vi "LVClass_Camera get Parameter Values OnlyGet.vi"(0 "Camera in":refnum<class "Camera.lvclass">, 11 "error in (no error)":errorcluster) -> (4 "Camera out":refnum<class "Camera.lvclass">, 6 "ListOfGettableValue":T1[](array[typedef]), 15 "error out":errorcluster)   [LabVIEW 2020, in "Camera.lvclass"]
doc: "Get camera parameters which are only gettable parameter \n\n<B>CameraIn</B> : Camera object.\n<B>CameraOut</B> : Camera object.\n<B>ListOfGettableValue</B> : Array of the parameter with readen value from camera object."
uses:
  Camera.lvclass
  CameraParametersSetup.ctl
  CameraParameters_Type.ctl
  Camera.lvclass/Camera.ctl
  LVClass_Camera Read acquisition state.vi
  LVClass_Camera Read all camera parameters.vi
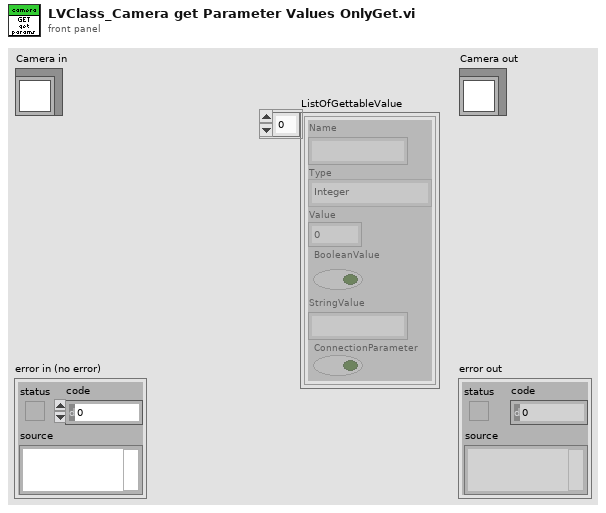
[diagram p1: front panel]
types:
  T1 = typedef "CameraParametersSetup.ctl" = cluster{"Name":string, "Type":T2, "Value":dbl, "BooleanValue":bool, "StringValue":string, "ConnectionParameter":bool}
  T2 = typedef "CameraParameters_Type.ctl" = enum16{"Integer", "Real", "String", "Boolean"}
  T3 = typedef "CameraAcquisitionState.ctl" = enum16{"Stop", "Live"}
  T4 = typedef "ParameterID.ctl" = cluster{"Name":string, "ConnectionParameter?":bool, "Type":T2, "Authorization":T5, "OnFlyAuthorization":T6, "StringValue":string, "Value":dbl, "Min":dbl, "Max":dbl, "BooleanValue":bool, "StringParameterList":string[]}
  T5 = typedef "CameraParameters_Authorization.ctl" = enum16{"Disable", "Gettable", "Settable - Gettable"}
  T6 = typedef "CameraParameters_OnFlyAuthorization.ctl" = enum16{"None", "Gettable", "Settable", "Settable - Gettable"}
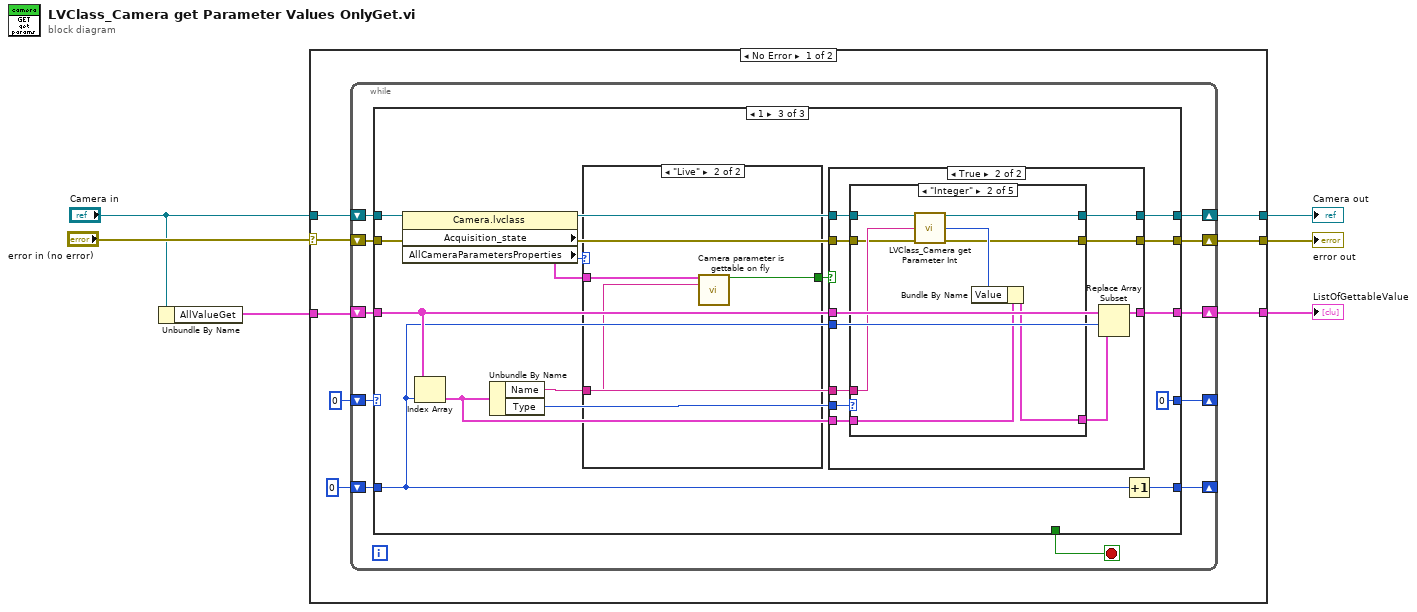
[diagram p0: block diagram]
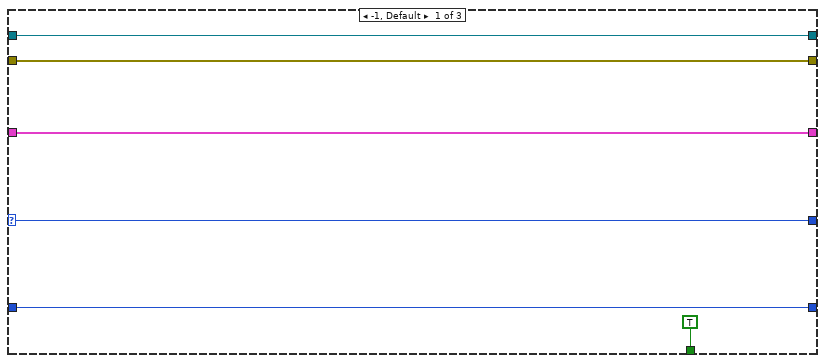
[diagram p2: hidden frame]
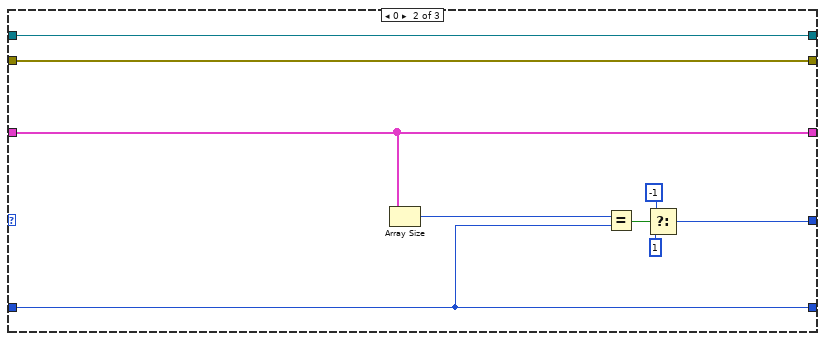
[diagram p3: hidden frame]
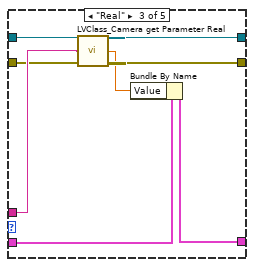
[diagram p6: hidden frame]
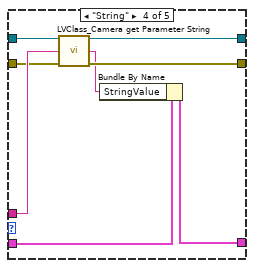
[diagram p7: hidden frame]
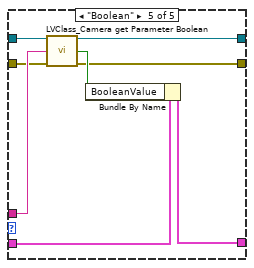
[diagram p8: hidden frame]
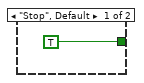
[diagram p9: hidden frame]
diagram:
  n1 = Unbundle By Name("Camera in") -> ("AllValueGet"=w1:T1[])
  n2 = case shown="No Error" "error in (no error)" {
    selector: "error in (no error)" -> [w10 w112]
    tunnel: [w11 w112] -> w5
    tunnel: [w12 w111] -> w4
    tunnel: "Camera in" -> [w14 w111]
    tunnel: [w9 _] -> w3
    tunnel: w1 -> [w7 _]
    frame No Error {
      n3 = while {
        shift-right: [w24] -> _
        shift-left: 0 -> [w23]
        shift-right: [w21] -> w11
        shift-left: w10 -> [w20]
        shift-right: [w22] -> w12
        shift-left: w14 -> [w25]
        shift-right: [w18] -> w9
        shift-left: w7 -> [w17]
        shift-right: [w15] -> _
        shift-left: 0 -> [w16]
        stop <- w19 stop-if-true
        n4 = case shown="1" w23 {
          selector: w23 -> [w26 _ _]
          tunnel: w25 -> [w30 w40 w48]
          tunnel: w20 -> [w29 w39 w46]
          tunnel: [w26 w33 0] -> w24
          tunnel: [w30 w40 w56] -> w22
          tunnel: [w29 w39 w55] -> w21
          tunnel: [TRUE _ _] -> w19
          tunnel: [w28 w38 w50] -> w18
          tunnel: w17 -> [w28 w38 w52]
          tunnel: w16 -> [w27 w36 w51]
          tunnel: [w27 w36 w54] -> w15
          frame -1, Default {
          }
          frame 0 {
            n5 = Array Size(array=w38) -> (size(s)=w37:i32)
            n6 = Equal?(x=w37, y=w36) -> (x = y?=w35:bool)
            n7 = Select(t=-1, s=w35, f=1) -> (s? t:f=w33:i32)
          }
          frame 1 {
            n8 = property class="Camera.lvclass"(reference=w48, error in=w46) -> (reference out=w47:refnum<class "Camera.lvclass">, error out=w45:errorcluster, "Acquisition_state"=w44:T3, "AllCameraParametersProperties"=w43:T4[])
            n9 = Index Array(array=w52, index=w51) -> (element=w53:T1)
            n10 = Unbundle By Name(w53) -> ("Name"=w41:string, "Type"=w49:T2)
            n11 = case shown="\"Live\"" w44 {
              tunnel: w43 -> [_ w109]
              tunnel: [TRUE w110] -> w42
              tunnel: w41 -> [_ w108]
              frame "Stop", Default {
              }
              frame "Live" {
                n12 = call "Camera parameter is gettable on fly.vi"("AllCameraParameters"=w109, "Name"=w108) -> ("Gettable?"=w110:bool)  [unwired: 13 in]
              }
            }
            n13 = case shown="True" w42 {
              tunnel: [w60 w71] -> w56
              tunnel: [w59 w70] -> w55
              tunnel: w53 -> [_ w69]
              tunnel: w52 -> [w58 w68]
              tunnel: w51 -> [_ w67]
              tunnel: [w58 w66] -> w50
              tunnel: w49 -> [_ w65]
              tunnel: w41 -> [_ w64]
              tunnel: w47 -> [w60 w63]
              tunnel: w45 -> [w59 w62]
              frame False {
              }
              frame True {
                n14 = case shown="\"Integer\"" w65 {
                  tunnel: w69 -> [w72 w82 w83 w91 w100]
                  tunnel: [w72 w81 w84 w98 w99] -> w61
                  tunnel: w64 -> [_ w80 w89 w95 w105]
                  tunnel: w63 -> [w74 w79 w90 w97 w106]
                  tunnel: [w74 w78 w86 w96 w103] -> w71
                  tunnel: [w73 w76 w87 w93 w101] -> w70
                  tunnel: w62 -> [w73 w75 w88 w94 w104]
                  frame Default {
                  }
                  frame "Integer" {
                    n15 = call "LVClass_Camera get Parameter Int.vi"("Camera in"=w79, "parameter_name"=w80, "error in (no error)"=w75) -> ("Camera out"=w78:refnum<class "Camera.lvclass">, "value"=w77:i32, "error out"=w76:errorcluster)  [unwired: 10 in]
                    n16 = Bundle By Name(cluster=w82, "Value"=w77) -> (w81:T1)
                  }
                  frame "Real" {
                    n17 = call "LVClass_Camera get Parameter Real.vi"("Camera in"=w90, "parameter_name"=w89, "error in (no error)"=w88) -> ("Camera out"=w86:refnum<class "Camera.lvclass">, "value"=w85:dbl, "error out"=w87:errorcluster)  [unwired: 10 in]
                    n18 = Bundle By Name(cluster=w83, "Value"=w85) -> (w84:T1)
                  }
                  frame "String" {
                    n19 = call "LVClass_Camera get Parameter String.vi"("Camera in"=w97, "parameter_name"=w95, "error in (no error)"=w94) -> ("Camera out"=w96:refnum<class "Camera.lvclass">, "value"=w92:string, "error out"=w93:errorcluster)  [unwired: 10 in]
                    n20 = Bundle By Name(cluster=w91, "StringValue"=w92) -> (w98:T1)
                  }
                  frame "Boolean" {
                    n21 = call "LVClass_Camera get Parameter Boolean.vi"("Camera in"=w106, "parameter_name"=w105, "error in (no error)"=w104) -> ("Camera out"=w103:refnum<class "Camera.lvclass">, "value"=w102:bool, "error out"=w101:errorcluster)  [unwired: 10 in]
                    n22 = Bundle By Name(cluster=w100, "BooleanValue"=w102) -> (w99:T1)
                  }
                }
                n23 = Replace Array Subset(array=w68, new element=w61, index=w67) -> (w66:T1[])
              }
            }
            n24 = Increment(x=w51) -> (x+1=w54:i32)
          }
        }
      }
    }
    frame Error {
    }
  }
  "error out" <- w5
  "Camera out" <- w4
  "ListOfGettableValue" <- w3
